vi "ReadBAESdataFromFileVer3.vi"(1 "Factor Size Parameter":dbl=1.0, 2 "Factor Extinction":dbl=1.0 min=0.0 max=150.0 step=1.0, 3 "Factor Ext Uncertainty":dbl=1.0 min=0.0 max=150.0 step=1.0, 4 "file path":path) -> (0 "Extinction ExtinctionUncertainity Size parameter and Number ofS sizes":T1)   [LabVIEW 2011]
uses:
  ReadBaesDataTypeDefinition.ctl
  <vilib>/Platform/storage/lvStorage.llb/_openStorageWithRootAutoDetect.vi
  <vilib>/Platform/storage/lvStorage.llb/xStorage/xStorageSupp/ErrorOut.vi
  <vilib>/Platform/storage/lvStorage.llb/_queryPropDateTime.vi
  <vilib>/Platform/storage/lvStorage.llb/_queryGenericObjects.vi
  <vilib>/Platform/storage/lvStorage.llb/_loadAllDouble.vi
  <vilib>/Platform/storage/Storage.llb/Get Object Info.vi
  <vilib>/Platform/storage/Storage.llb/__closeStorageFromObject.vi
  <vilib>/imath/engines/lvmath2/RunTimeEngine/ErrorHandling/NIMS_Finalize Error.vi
  <vilib>/imath/engines/lvmath2/RunTimeEngine/Managers/WorkSpace/UID Generator.vi
  <vilib>/imath/engines/lvmath2/RunTimeEngine/VariableToken/Read/NIMS_Get Elements - SorM(_,$) - Check.vi
  <instcachedir>/0/NIMS_Get Elements - SorM(_,$) - Check_3B494CC2A76E49EA8E6F8F732E2632C3.lvgen/NIMS_Get Elements - SorM(_,$) - Check_3B494CC2A76E49EA8E6F8F732E2632C3_000.vi
  <vilib>/imath/engines/lvmath2/RunTimeEngine/BuiltInFunctions/length/NIMS_length(GV).vi
  <instcachedir>/0/NIMS_length(GV)_08A3D13377FD4E4B96F5795FBF3698FA.lvgen/NIMS_length(GV)_08A3D13377FD4E4B96F5795FBF3698FA_000.vi
  <vilib>/imathl/engines/lvmath/Functions/Error Handling/Create Error.vi
  <vilib>/imath/engines/lvmath2/RunTimeEngine/Managers/SymbolTable/Clear UID.vi
  <vilib>/imath/engines/lvmath2/RunTimeEngine/NodeEndStatement/NIMS_NodeEndStatement_Output.vi
  <instcachedir>/0/NIMS_NodeEndStatement_Output_53EC0D466D134D7ABD903AC30B43404B.lvgen/NIMS_NodeEndStatement_Output_53EC0D466D134D7ABD903AC30B43404B_005.vi
  <instcachedir>/0/NIMS_NodeEndStatement_Output_53EC0D466D134D7ABD903AC30B43404B.lvgen/NIMS_NodeEndStatement_Output_53EC0D466D134D7ABD903AC30B43404B_001.vi
  <instcachedir>/0/NIMS_NodeEndStatement_Output_53EC0D466D134D7ABD903AC30B43404B.lvgen/NIMS_NodeEndStatement_Output_53EC0D466D134D7ABD903AC30B43404B_002.vi
  <vilib>/imath/engines/lvmath2/RunTimeEngine/RangeToken/NIMS_Range.vi
  <instcachedir>/0/NIMS_Range_0B7635FB69F84E19AA68E7FF959DF37C.lvgen/NIMS_Range_0B7635FB69F84E19AA68E7FF959DF37C_001.vi
  <vilib>/imath/engines/lvmath2/RunTimeEngine/VariableToken/Read/NIMS_Get Elements - SorM(_,_) - Check - Check(_).vi
  <instcachedir>/0/NIMS_Get Elements - SorM(_,_) - Check - Check(_)_B78B880141DE464ABBC753BC43E627FC.lvgen/NIMS_Get Elements - SorM(_,_) - Check - Check(_)_B78B880141DE464ABBC753BC43E627FC_009.vi
  <vilib>/imath/engines/lvmath2/RunTimeEngine/ErrorHandling/NIMS_Create Error From Enums.vi
  <vilib>/imath/engines/lvmath2/RunTimeEngine/RangeToken/NIMS_Range_R2.vi
  <vilib>/imath/engines/lvmath2/RunTimeEngine/VariableToken/Read/NIMS_Get Elements - SorM(_,_) - Check - Check.vi
  <instcachedir>/0/NIMS_Get Elements - SorM(_,_) - Check - Check_DA1E252EAB634D989357E7C72E8137F5.lvgen/NIMS_Get Elements - SorM(_,_) - Check - Check_DA1E252EAB634D989357E7C72E8137F5_006.vi
  <vilib>/imath/engines/lvmath2/RunTimeEngine/BuiltInFunctions/repeatmx/NIMS_repeatmx(GM, I32, I32).vi
  <instcachedir>/0/NIMS_repeatmx(GM, I32, I32)_8C2ED2EBCBCE41FC8E83AC0E124C0986.lvgen/NIMS_repeatmx(GM, I32, I32)_8C2ED2EBCBCE41FC8E83AC0E124C0986_000.vi
  <vilib>/imath/engines/lvmath2/RunTimeEngine/ArithmeticOperatorToken/NIMS_ArithmeticOperator_rightdiv.vi
  <instcachedir>/0/NIMS_ArithmeticOperator_rightdiv_85C5B8074732470A99000A2C3876C445.lvgen/NIMS_ArithmeticOperator_rightdiv_85C5B8074732470A99000A2C3876C445_004.vi
  <vilib>/imath/engines/lvmath2/RunTimeEngine/RunTimeType/NIMS_RunTimeType_From StrictType (excl LVString).vi
  <instcachedir>/0/NIMS_RunTimeType_From StrictType (excl LVString)_46AE8B54A11948F0BCCEB8091EE7AA4C.lvgen/NIMS_RunTimeType_From StrictType (excl LVString)_46AE8B54A11948F0BCCEB8091EE7AA4C_000.vi
  <vilib>/imath/engines/lvmath2/RunTimeEngine/LocalVariableDefStatement/MC_LocalVariableDefStatement_Display.vi
  <instcachedir>/0/NIMS_Get Elements - SorM(_,_) - Check - Check(_)_B78B880141DE464ABBC753BC43E627FC.lvgen/NIMS_Get Elements - SorM(_,_) - Check - Check(_)_B78B880141DE464ABBC753BC43E627FC_010.vi
  <vilib>/Platform/storage/lvStorage.llb/xStorage/Open Data Storage/Open Data Storage.xnode
  <vilib>/Platform/storage/lvStorage.llb/xStorage/Read Data/Read Data.xnode
  <vilib>/Platform/storage/lvStorage.llb/xStorage/Close Data Storage/Close Data Storage.xnode
  <vilib>/imath/engines/lvmath2/RunTimeEngine/Managers/SymbolTable/NIMS_WorkSpace.lvlib
panel:
  out "WaveLengths 2":dbl[](array[numeric])
  out "Sizes":dbl[](array[numeric])
  in  "Extinction ExtinctionUncertainity Size parameter and Number ofS sizes 2":T1
  out "Signal":dbl[][](array[numeric])
  out "GeometricCrossSection":dbl[](array[numeric])
  out "Number Of Sizes":dbl
  out "SizeParameter":dbl[][](array[numeric])
  in  "Slide":i16(slide) scale=0.0..100.0
  out "Extinction Graph":cluster{"Extinction":dbl[], "Sizes":dbl[]}[](graph)
  out "ExtinctionUncertainty":dbl[][](array[numeric])
  out "Extinction":dbl[][](array[numeric])
  out "WaveLengths":dbl[](array[numeric])
  out "error out":errorcluster
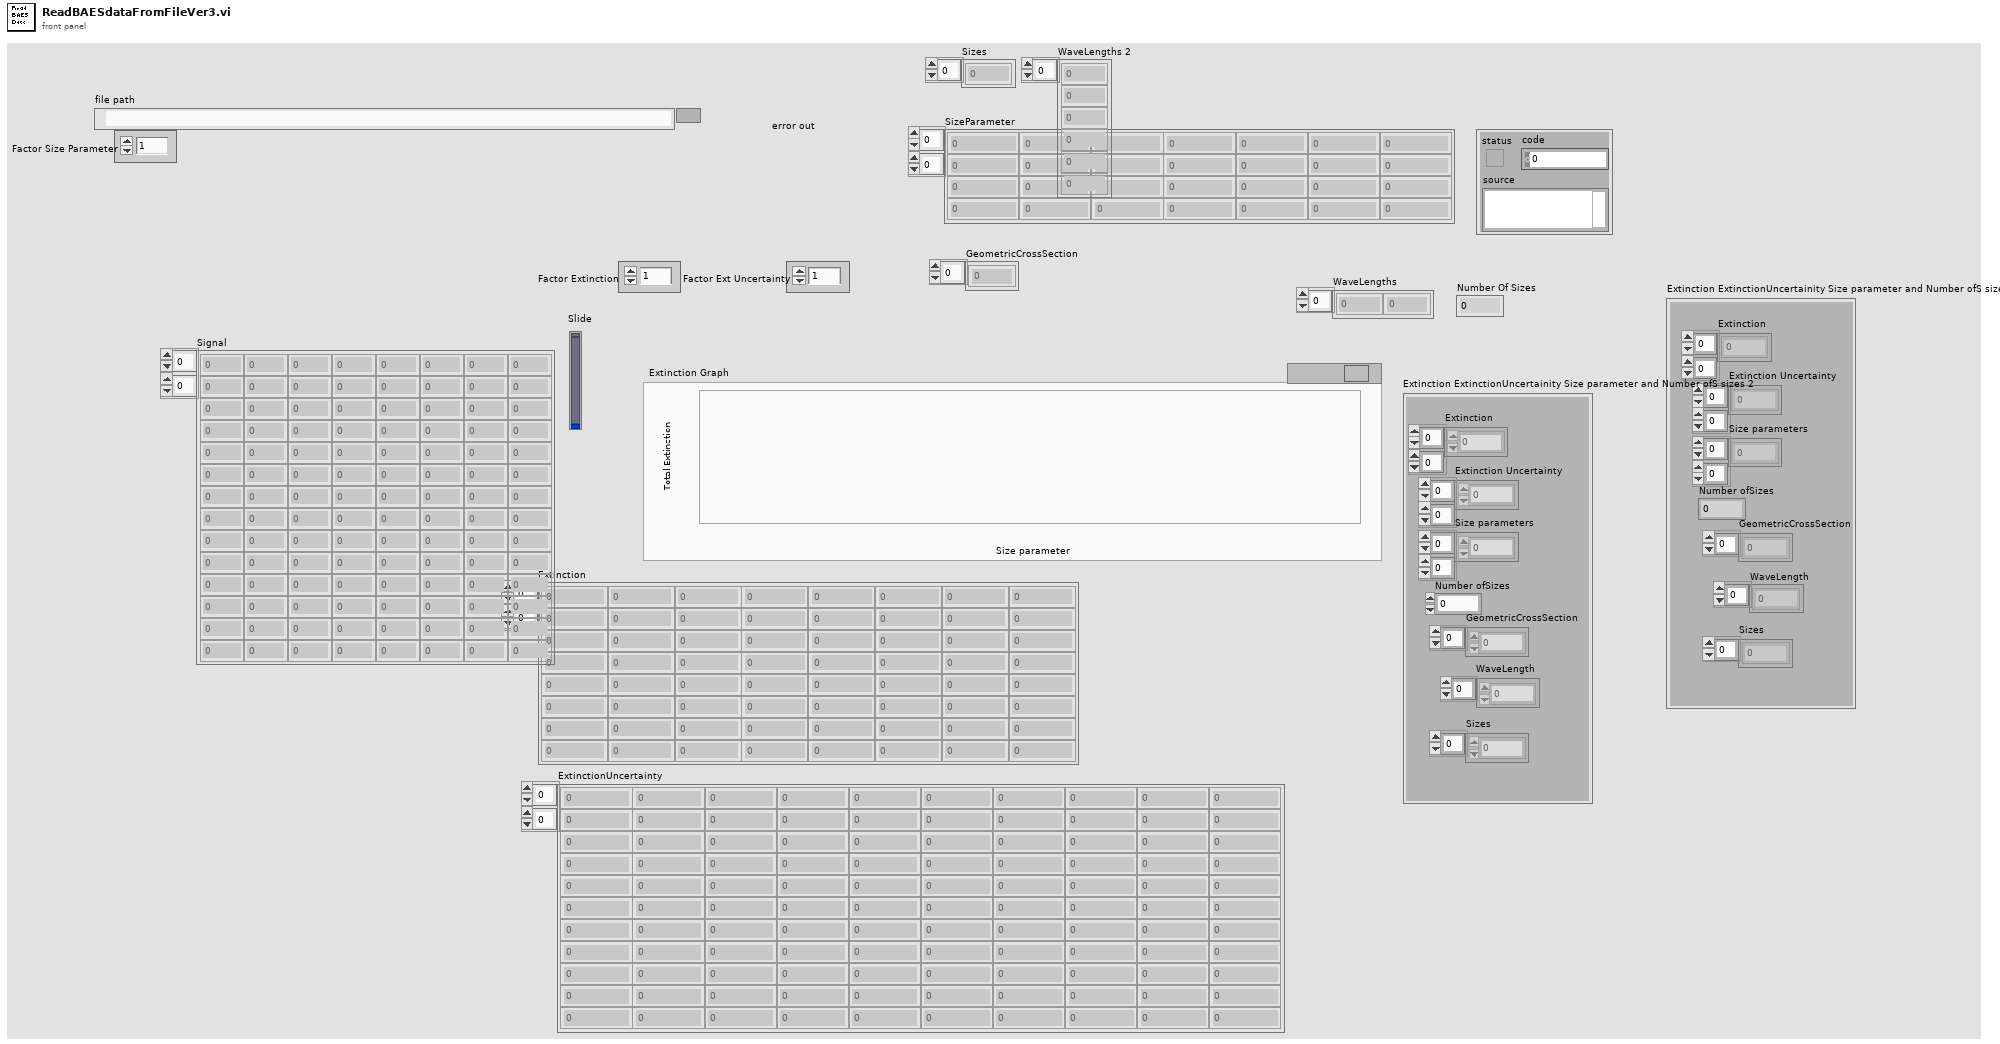
[diagram p1: front panel]
types:
  T1 = typedef "ReadBaesDataTypeDefinition.ctl" = cluster{"Extinction":dbl[][], "Extinction Uncertainty":dbl[][], "Size parameters":dbl[][], "Number ofSizes":dbl, "GeometricCrossSection":dbl[], "WaveLength":dbl[], "Sizes":dbl[]}
  T2 = enum16{"open", "open or create", "create or replace", "create", "open (read only)"}
  T3 = cluster{"SizeParameter":dbl[], "Extinction":dbl[]}
  T4 = cluster{"SizeParameter":dbl[], "Extinction":dbl[]}[]
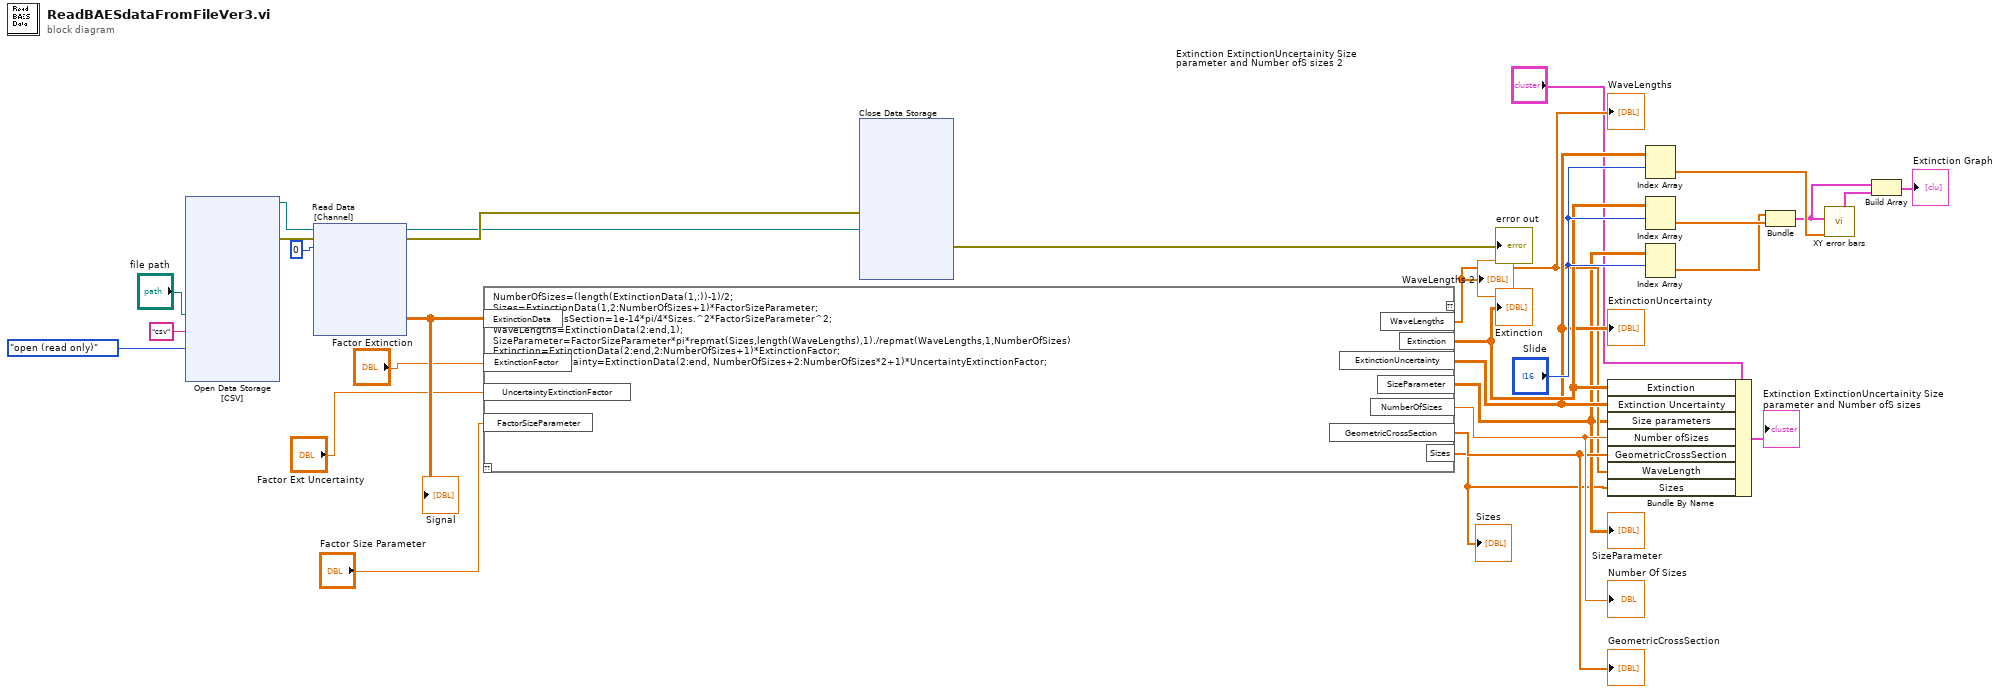
[diagram p0: block diagram]
diagram:
  n1 = xnode "Open Data Storage\n[CSV]"("file path"="file path", "DataPlugin name"="csv", "function (open:0)"=T2."open (read only)") -> ("storage refnum (file)"=w29:refnum<k20>, "error out"=w28:errorcluster)  [unwired: 2 in, 1 out]
  n2 = xnode "Read Data\n[Channel]"("storage refnum (file)"=w29, "error in"=w28, "index"=0) -> ("Signal"=w15:dbl[][], "storage refnum (file) out"=w23:refnum<k20>, "error out"=w27:errorcluster)  [unwired: 1 in, 1 out]
  "Signal" <- w15
  n3 = mathscript code="NumberOfSizes=(length(ExtinctionData(1,:))-1)/2;\nSizes=ExtinctionData(1,2:NumberOfSizes+1)*FactorSizeParameter;\nGeometricCrossSection=1e-14*pi/4*Sizes.^2*FactorSizeParameter^2;\nWaveLengths=ExtinctionData(2:end,1);\nSizeParameter=FactorSizeParameter*pi*repmat(Sizes,length(WaveLengths),1)./repmat(WaveLengths,1,NumberOfSizes)\nExtinction=ExtinctionData(2:end,2:NumberOfSizes+1)*ExtinctionFactor;\nExtinctionUncertainty=ExtinctionData(2:end, NumberOfSizes+2:NumberOfSizes*2+1)*UncertaintyExtinctionFactor;"("ExtinctionData"=w15, "ExtinctionFactor"="Factor Extinction", "UncertaintyExtinctionFactor"="Factor Ext Uncertainty", "FactorSizeParameter"="Factor Size Parameter") -> ("WaveLengths"=w8:dbl[], "Extinction"=w12:dbl[][], "ExtinctionUncertainty"=w11:dbl[][], "SizeParameter"=w7:dbl[][], "NumberOfSizes"=w10:dbl, "GeometricCrossSection"=w9:dbl[], "Sizes"=w4:dbl[])  [unwired: 1 in, 1 out]
  "WaveLengths" <- w8
  "Extinction" <- w12
  "ExtinctionUncertainty" <- w11
  "SizeParameter" <- w7
  "Number Of Sizes" <- w10
  "GeometricCrossSection" <- w9
  "Sizes" <- w4
  "WaveLengths 2" <- w8
  n4 = xnode "Close Data Storage\n"("error in (no error)"=w27, "storage refnum (file)"=w23) -> ("error out"=→"error out":errorcluster)  [unwired: 1 out]
  n5 = Bundle By Name(cluster="Extinction ExtinctionUncertainity Size parameter and Number ofS sizes 2", "Extinction"=w12, "Extinction Uncertainty"=w11, "Size parameters"=w7, "Number ofSizes"=w10, "GeometricCrossSection"=w9, "WaveLength"=w8, "Sizes"=w4) -> (→"Extinction ExtinctionUncertainity Size parameter and Number ofS sizes":T1)
  n6 = Index Array(array=w11, index (row)="Slide") -> (element=w22:dbl[])  [unwired: 1 in]
  n7 = Index Array(array=w12, index (row)="Slide") -> (element=w18:dbl[])  [unwired: 1 in]
  n8 = Index Array(array=w7, index (row)="Slide") -> (element=w16:dbl[])  [unwired: 1 in]
  n9 = Bundle("SizeParameter"=w16, "Extinction"=w18) -> (w21:T3)  [unwired: 1 in]
  n10 = call "XY error bars.vi"("XY plot"=w21, "Yerror"=w22) -> ("Y error bars"=w20:cluster{dbl[], dbl[]})  [unwired: 6 in, 2 out]
  n11 = Build Array(w21, w20) -> (→"Extinction Graph":T4)
